vi "Main.vi"() -> ()   [LabVIEW 2018] (continued)
            n155 = Decimal String To Number(string=w532, default (0L)=u32 0 ("默认(0 I32)")) -> (number=w538:u32)  [unwired: 1 in, 1 out]
            n156 = call "S7_Write.vi"("TCP"=w537, "寄存器类型"=w541, "DB #"=u16 20, "写入地址"=u32 58, "数据类型"=w542, "写入数据"=w538) -> ("TCP"=w534:refnum<k5>, "error out"=w533:errorcluster)  [unwired: 7 in, 1 out]
            n157 = Bundle By Name(cluster=w545, "数据保存超时"=w532) -> (w544:T5)
          }
          frame "------------" {
          }
          frame "错误" {
            n158 = Flush Queue(queue=w556) -> ()  [unwired: 1 in, 3 out]
            n159 = Flush Queue(queue=w555) -> ()  [unwired: 1 in, 3 out]
            n160 = call "S7_Close.vi"("TCP Connection Ref"=w559) -> ("error out"=w557:errorcluster)  [unwired: 10 in]
            n161 = call <vilib>:"Clear Errors.vi"("error in (no error)"=w557) -> ()  [unwired: 5 in, 2 out]
          }
          frame "退出" {
            n162 = Release Queue(queue=w567) -> ()  [unwired: 2 in, 3 out]
            n163 = Release Queue(queue=w566) -> ()  [unwired: 2 in, 3 out]
            n164 = call "S7_Close.vi"("TCP Connection Ref"=w565) -> ("error out"=w562:errorcluster)  [unwired: 10 in]
          }
          frame "看门狗" {
            w582 = u8 132 items=["I/O (P)"=128, "Input (I)"=129, "Output (Q)"=130, "Bit Memory (M)"=131, "Data (DB)"=132, "Instance Data (DI)"=133, "Local Data (L)"=134, "Predecessor Local Data (VL)"=135] ("寄存器类型")
            w583 = u16 1 items=["byte", "word", "Dword"] ("数据类型")
            n165 = Unbundle By Name(w575) -> ("看门狗"=w585:string)
            n166 = Decimal String To Number(string=w585) -> (number=w586:i32)  [unwired: 2 in, 1 out]
            n167 = Equal?(x=w586, y=0) -> (x = y?=w588:bool)
            n168 = case shown="假" w588 {
              tunnel: [0 ("y") 1 ("y")] -> w576
              frame False {
              }
              frame True {
              }
            }
            "80" <- w576
            n169 = call "S7_Write.vi"("TCP"=w580, "寄存器类型"=w582, "DB #"=u16 20, "写入地址"=u32 8, "数据类型"=w583, "写入数据"=w576) -> ("TCP"=w573:refnum<k5>, "error out"=w571:errorcluster)  [unwired: 7 in, 1 out]
            n170 = Number To Decimal String(number=w576) -> (decimal integer string=w577:string)  [unwired: 1 in]
            n171 = Bundle By Name(cluster=w575, "看门狗"=w577) -> (w574:T5)
            n172 = disable-structure shown="启用" {
              disable-tunnel: w573 -> [w589 w605]
              disable-tunnel: [w589 w597] -> w572
              disable-tunnel: w571 -> [w590 w596]
              disable-tunnel: [w590 w594] -> w570
              frame Disabled {
              }
              frame Enabled {
                w603 = u16 20 ("DB #")
                w602 = u8 132 items=["I/O (P)"=128, "Input (I)"=129, "Output (Q)"=130, "Bit Memory (M)"=131, "Data (DB)"=132, "Instance Data (DI)"=133, "Local Data (L)"=134, "Predecessor Local Data (VL)"=135] ("寄存器类型")
                w601 = u16 1 items=["byte", "word", "Dword"] ("数据类型")
                n173 = call "S7_Read.vi"("TCP"=w605, "DB #"=w603, "读取长度"=u16 1, "寄存器类型"=w602, "起始地址"=u32 48 ("写入地址"), "数据类型"=w601, "error in"=w596) -> ("TCP"=w604:refnum<k5>, "数据"=w598:u32[], "error out"=w595:errorcluster)  [unwired: 5 in, 1 out]
                n174 = Index Array(array=w598) -> (element=w592:u32)  [unwired: 1 in]
                "80产品型号" <- w592
                n175 = case shown="2" w592 {
                  tunnel: ["未选择" "1" "2"] -> w591
                  frame 0, Default {
                  }
                  frame 1 {
                  }
                  frame 2 {
                  }
                }
                "产品型号" <- w591
                n176 = call "S7_Write.vi"("TCP"=w604, "寄存器类型"=w602, "DB #"=w603, "写入地址"=u32 50, "数据类型"=w601, "写入数据"=w592, "error in"=w595) -> ("TCP"=w597:refnum<k5>, "error out"=w594:errorcluster)  [unwired: 6 in, 1 out]
              }
            }
          }
        }
      }
      n177 = while {
        shift-right: [w6079] -> _
        shift-left: cluster{"Data":string[], "State":T1} {"Data"=[], "State"=enum."PLC通讯初始化"} ("元素") -> [w6080]
        shift-right: [w6088] -> _
        shift-left: w135 -> [w6085]
        shift-right: [w6089] -> _
        shift-left: _ -> [w6086]
        tunnel: w109 -> [w6081]
        tunnel: w116 -> [w6076]
        tunnel: w134 -> [_]
        shift-right: [w6075] -> _
        shift-left: _ -> [w6074]
        stop <- w6077 stop-if-true
        # "OP70"
        n178 = local read "退出"() -> (w6084:bool)
        n179 = Wait (ms)(milliseconds to wait=u32 20 ("等待时间（毫秒）")) -> ()  [unwired: 1 out]
        n180 = call "状态判断.vi"("error IO"=w6085, "退出？"=w6084, "簇 输入"=w6080, "队列输入"=w6081) -> ("簇"=w6083:cluster{"Data":string[], "State":T1})  [unwired: 6 in, 1 out]
        n181 = Unbundle By Name(w6083) -> ("Data"=w6078:string[], "State"=w6082:T1)
        "70_State" <- w6082
        n182 = case shown="\"退出\"" w6082 {
          tunnel: [w6093 w6120 w6142 w6173 w6194 w6245 w6265 w6374 w6402 w6417 refnum<k5> refnum ("TCP") refnum<k5> refnum ("TCP") w6437] -> w6089
          tunnel: [w6094 errorcluster {"status"=FALSE, "code"=0, "source"=""} ("error out") w6141 w6169 w6193 errorcluster {"status"=FALSE, "code"=0, "source"=""} ("error out") w6264 w6321 w6403 errorcluster {"status"=FALSE, "code"=0, "source"=""} ("error out") errorcluster {"status"=FALSE, "code"=0, "source"=""} ("error out") w6429 w6435] -> w6088
          tunnel: w6086 -> [_ w6120 w6143 w6174 w6195 w6245 w6266 w6305 w6405 w6417 w6423 w6430 w6462]
          tunnel: w6081 -> [w6106 _ w6124 _ _ _ w6246 _ _ _ w6419 w6431 _]
          tunnel: [cluster{"Data":string[], "State":T1} {"Data"=[], "State"=enum."读扫码请求"} ("元素") cluster{"Data":string[], "State":T1} {"Data"=[], "State"=enum."读扫码请求"} ("元素") w6131 cluster{"Data":string[], "State":T1} {"Data"=[], "State"=enum."读数据保存请求"} ("元素") cluster{"Data":string[], "State":T1} {"Data"=[], "State"=enum."读数据保存请求"} ("元素") cluster{"Data":string[], "State":T1} {"Data"=[], "State"=enum."读数据保存请求"} ("元素") w6254 cluster{"Data":string[], "State":T1} {"Data"=[], "State"=enum."看门狗"} ("元素") cluster{"Data":string[], "State":T1} {"Data"=[], "State"=enum."看门狗"} ("元素") cluster{"Data":string[], "State":T1} {"Data"=[], "State"=enum."看门狗"} ("元素") cluster{"Data":string[], "State":T1} {"Data"=[], "State"=enum."PLC通讯初始化"} ("元素") cluster{"Data":string[], "State":T1} {"Data"=[], "State"=enum."退出"} ("元素") cluster{"Data":string[], "State":T1} {"Data"=[], "State"=enum."读扫码请求"} ("元素")] -> w6079
          tunnel: w6078 -> [_ _ _ _ w6191 _ _ _ w6404 _ _ _ _]
          tunnel: [FALSE FALSE FALSE FALSE FALSE FALSE FALSE FALSE FALSE FALSE FALSE TRUE FALSE] -> w6077
          tunnel: w6076 -> [_ _ _ _ _ _ _ w6381 _ _ w6420 w6432 _]
          tunnel: [T10 {"扫码超时"="999", "数据保存超时"="999", "看门狗"="999"} w6116 w6123 w6170 w6189 w6241 w6247 w6371 w6398 w6413 w6418 w6427 w6456] -> w6075
          tunnel: w6074 -> [_ w6116 w6123 w6170 w6190 w6241 w6247 w6371 w6399 w6413 w6418 w6427 w6457]
          frame "PLC通讯初始化", Default {
            w6099 = u16 0 items=["byte", "word", "Dword"] ("数据类型")
            w6103 = u8 132 items=["I/O (P)"=128, "Input (I)"=129, "Output (Q)"=130, "Bit Memory (M)"=131, "Data (DB)"=132, "Instance Data (DI)"=133, "Local Data (L)"=134, "Predecessor Local Data (VL)"=135] ("寄存器类型")
            w6114 = u8 0 items=["S7-1200.200.200SMART"=0, "S7-300"=2, "S7-400"=3] ("PLC 系列")
            n183 = Enqueue Element(queue=w6106, element=cluster{"Data":string[], "State":T1} {"Data"=["999"], "State"=enum."扫码回复"} ("元素")) -> (queue out=w6110:refnum<queue>, error out=w6109:errorcluster)  [unwired: 2 in, 1 out]
            n184 = call "S7_Open.vi"("IP 地址"="192.168.0.70", "PLC 系列"=w6114, "超时（MS）"=100) -> ("TCP"=w6096:refnum<k5>, "error out"=w6095:errorcluster)  [unwired: 10 in, 1 out]
            n185 = Unbundle By Name(w6095) -> ("status"=→"ST70通讯状态":bool)
            n186 = Enqueue Element(queue=w6110, element=cluster{"Data":string[], "State":T1} {"Data"=["999"], "State"=enum."数据保存回复"} ("元素"), error in (no error)=w6109) -> ()  [unwired: 1 in, 3 out]
            n187 = call "S7_Read.vi"("TCP"=w6096, "DB #"=u16 20, "读取长度"=u16 17, "寄存器类型"=w6103, "起始地址"=u32 38, "数据类型"=w6099, "error in"=w6095) -> ("TCP"=w6093:refnum<k5>, "数据"=w6098:u32[], "error out"=w6094:errorcluster)  [unwired: 5 in, 1 out]
            n188 = To Unsigned Word Integer(number=w6098) -> (unsigned 16bit integer=w6097:u16[])
            n189 = call "还原为字符串.vi"("输入数组"=w6097) -> ("字符串"=w6091:string)  [unwired: 9 in, 1 out]
            n190 = Match Pattern(string=w6091, regular expression=" " ("正则表达式")) -> (before substring=w6090:string)  [unwired: 1 in, 3 out]
            n191 = local write "70二维码"(w6090) -> ()
          }
          frame "--------------" {
          }
          frame "读扫码请求" {
            w6151 = u16 0 items=["byte", "word", "Dword"] ("数据类型")
            w6153 = u8 132 items=["I/O (P)"=128, "Input (I)"=129, "Output (Q)"=130, "Bit Memory (M)"=131, "Data (DB)"=132, "Instance Data (DI)"=133, "Local Data (L)"=134, "Predecessor Local Data (VL)"=135] ("寄存器类型")
            n192 = call "S7_Read.vi"("TCP"=w6143, "DB #"=u16 20, "读取长度"=u16 1, "寄存器类型"=w6153, "起始地址"=u32 0, "数据类型"=w6151) -> ("TCP"=w6142:refnum<k5>, "数据"=w6148:u32[], "读取成功"=w6121:bool, "error out"=w6141:errorcluster)  [unwired: 6 in]
            n193 = Not(x=w6121) -> (.not. x?=w6122:bool)
            n194 = local write "ST70通讯状态"(w6122) -> ()
            n195 = Index Array(array=w6148, index=0 ("索引")) -> (element=w6146:u32)
            n196 = Number To Boolean Array(number=w6146) -> (Boolean array=w6145:bool[])
            n197 = Index Array(array=w6145, index=0 ("索引")) -> (element=w6130:bool)
            "ST70扫码请求" <- w6130
            n198 = Unbundle By Name(w6123) -> ("扫码超时"=w6125:string)
            n199 = Not Equal?(x=w6125, y="999") -> (x != y?=w6127:bool)
            n200 = call <vilib>:"Boolean Crossing PtByPt.vi"("direction"=enum16{"either", "false-true", "true-false"}."false-true", "input"=w6130) -> ("crossing"=w6137:bool)  [unwired: 1 in]
            n201 = call <vilib>:"Boolean Crossing PtByPt.vi"("direction"=enum16{"either", "false-true", "true-false"}."true-false", "input"=w6130) -> ("crossing"=w6136:bool)  [unwired: 1 in]
            n202 = Not(x=w6127) -> (.not. x?=w6128:bool)
            n203 = call "已用时间15"("Reset"=w6128) -> ("Time has Elapsed"=w6129:bool)  [unwired: 11 in, 7 out]
            n204 = Insert Into Array(array=bool[] [] ("数组"), index=0 ("索引"), new element #1=w6137, new element #2=w6136) -> (w6133:bool[])
            n205 = Boolean Array To Number(Boolean array=w6133) -> (number=w6132:u32)
            n206 = case shown="1" w6132 {
              tunnel: [cluster{"Data":string[], "State":T1} {"Data"=[], "State"=enum."读数据保存请求"} ("元素") w6158 w6162] -> w6131
              tunnel: w6124 -> [_ w6159 w6163]
              frame 0, Default {
              }
              frame 1 {
                w6158 = cluster{"Data":string[], "State":T1} {"Data"=[], "State"=enum."读二维码"} ("元素")
                n207 = Enqueue Element(queue=w6159, element=w6158, timeout in ms (-1)=10 ("超时毫秒(-1)")) -> ()  [unwired: 1 in, 3 out]
              }
              frame 2 {
                w6162 = cluster{"Data":string[], "State":T1} {"Data"=["999"], "State"=enum."扫码回复"} ("元素")
                n208 = Enqueue Element(queue=w6163, element=w6162, timeout in ms (-1)=10 ("超时毫秒(-1)")) -> ()  [unwired: 1 in, 3 out]
              }
            }
            n209 = case shown="真" w6129 {
              tunnel: w6124 -> [_ w6155]
              frame False {
              }
              frame True {
                n210 = Enqueue Element(queue=w6155, element=cluster{"Data":string[], "State":T1} {"Data"=["999"], "State"=enum."扫码回复"} ("元素"), timeout in ms (-1)=10 ("超时毫秒(-1)")) -> ()  [unwired: 1 in, 3 out]
              }
            }
          }
          frame "读二维码" {
            w6179 = u16 0 items=["byte", "word", "Dword"] ("数据类型")
            w6175 = u8 132 items=["I/O (P)"=128, "Input (I)"=129, "Output (Q)"=130, "Bit Memory (M)"=131, "Data (DB)"=132, "Instance Data (DI)"=133, "Local Data (L)"=134, "Predecessor Local Data (VL)"=135] ("寄存器类型")
            n211 = call "S7_Read.vi"("TCP"=w6174, "DB #"=u16 20, "读取长度"=u16 17, "寄存器类型"=w6175, "起始地址"=u32 38, "数据类型"=w6179) -> ("TCP"=w6173:refnum<k5>, "数据"=w6180:u32[], "error out"=w6182:errorcluster)  [unwired: 6 in, 1 out]
            n212 = To Unsigned Word Integer(number=w6180) -> (unsigned 16bit integer=w6181:u16[])
            n213 = call "还原为字符串.vi"("error in (no error)"=w6182, "输入数组"=w6181) -> ("error out"=w6166:errorcluster, "字符串"=w6167:string)  [unwired: 8 in]
            n214 = Match Pattern(string=w6167, regular expression=" " ("正则表达式")) -> (before substring=w6164:string)  [unwired: 1 in, 3 out]
            n215 = flat-sequence {
              tunnel: w6166 -> [w6184]
              tunnel: [w6184] -> w6165
              tunnel: w6164 -> [w6183]
              tunnel: [w6186] -> w6169
              tunnel: w6165 -> [w6185]
              frame #0 {
                "70二维码" <- w6183
              }
              frame #1 {
                n216 = property on="ST70扫码请求(事件)" class="Bool (严格)"(error in=w6185, "Val(Sgnl)"=TRUE ("值(信号)")) -> (error out=w6186:errorcluster)  [unwired: 1 in, 1 out]
              }
            }
          }
          frame "扫码回复" {
            n217 = Array Size(array=w6191) -> (size(s)=w6192:i32)
            n218 = case shown="3, 默认" w6192 {
              tunnel: w6191 -> [w6200 w6233]
              tunnel: w6195 -> [w6199 w6220]
              tunnel: [w6201 w6211] -> w6194
              tunnel: [w6202 w6210] -> w6193
              tunnel: [w6198 w6209] -> w6188
              frame 1 {
                w6205 = u8 132 items=["I/O (P)"=128, "Input (I)"=129, "Output (Q)"=130, "Bit Memory (M)"=131, "Data (DB)"=132, "Instance Data (DI)"=133, "Local Data (L)"=134, "Predecessor Local Data (VL)"=135] ("寄存器类型")
                w6204 = u16 1 items=["byte", "word", "Dword"] ("数据类型")
                n219 = Index Array(array=w6200) -> (element=w6198:string)  [unwired: 1 in]
                n220 = Decimal String To Number(string=w6198, default (0L)=u32 0 ("默认(0 I32)")) -> (number=w6208:u32)  [unwired: 1 in, 1 out]
                n221 = call "S7_Write.vi"("TCP"=w6199, "寄存器类型"=w6205, "DB #"=u16 20, "写入地址"=u32 2, "数据类型"=w6204, "写入数据"=w6208) -> ("TCP"=w6201:refnum<k5>, "error out"=w6202:errorcluster)  [unwired: 7 in, 1 out]
              }
              frame 3, Default {
                w6223 = u8 132 items=["I/O (P)"=128, "Input (I)"=129, "Output (Q)"=130, "Bit Memory (M)"=131, "Data (DB)"=132, "Instance Data (DI)"=133, "Local Data (L)"=134, "Predecessor Local Data (VL)"=135] ("寄存器类型")
                w6222 = u16 1 items=["byte", "word", "Dword"] ("数据类型")
                w6230 = u8 132 items=["I/O (P)"=128, "Input (I)"=129, "Output (Q)"=130, "Bit Memory (M)"=131, "Data (DB)"=132, "Instance Data (DI)"=133, "Local Data (L)"=134, "Predecessor Local Data (VL)"=135] ("寄存器类型")
                w6231 = u16 1 items=["byte", "word", "Dword"] ("数据类型")
                w6237 = u8 132 items=["I/O (P)"=128, "Input (I)"=129, "Output (Q)"=130, "Bit Memory (M)"=131, "Data (DB)"=132, "Instance Data (DI)"=133, "Local Data (L)"=134, "Predecessor Local Data (VL)"=135] ("寄存器类型")
                w6236 = u16 1 items=["byte", "word", "Dword"] ("数据类型")
                n222 = Index Array(array=w6233) -> (element #1=w6209:string, element #2=w6216:string, element #3=w6215:string)  [unwired: 3 in]
                n223 = Equal?(x=w6215, y="OK") -> (x = y?=w6213:bool)
                n224 = Decimal String To Number(string=w6216, default (0L)=u32 0 ("默认(0 I32)")) -> (number=w6217:u32)  [unwired: 1 in, 1 out]
                n225 = case shown="假" w6213 {
                  tunnel: [u32 2 ("写入数据") u32 1 ("写入数据")] -> w6212
                  frame False {
                  }
                  frame True {
                  }
                }
                n226 = call "S7_Write.vi"("TCP"=w6220, "寄存器类型"=w6237, "DB #"=u16 20, "写入地址"=u32 8, "数据类型"=w6236, "写入数据"=w6217) -> ("TCP"=w6227:refnum<k5>, "error out"=w6228:errorcluster)  [unwired: 7 in, 1 out]
                n227 = call "S7_Write.vi"("TCP"=w6227, "寄存器类型"=w6230, "DB #"=u16 20, "写入地址"=u32 10, "数据类型"=w6231, "写入数据"=w6212, "error in"=w6228) -> ("TCP"=w6219:refnum<k5>, "error out"=w6218:errorcluster)  [unwired: 6 in, 1 out]
                n228 = Decimal String To Number(string=w6209, default (0L)=u32 0 ("默认(0 I32)")) -> (number=w6226:u32)  [unwired: 1 in, 1 out]
                n229 = call "S7_Write.vi"("TCP"=w6219, "寄存器类型"=w6223, "DB #"=u16 20, "写入地址"=u32 2, "数据类型"=w6222, "写入数据"=w6226, "error in"=w6218) -> ("TCP"=w6211:refnum<k5>, "error out"=w6210:errorcluster)  [unwired: 6 in, 1 out]
              }
            }
            "扫码请求回复70" <- w6188
            n230 = Bundle By Name(cluster=w6190, "扫码超时"=w6188) -> (w6189:T10)
          }
          frame "-------------" {
          }
          frame "读数据保存请求" {
            w6274 = u16 0 items=["byte", "word", "Dword"] ("数据类型")
            w6276 = u8 132 items=["I/O (P)"=128, "Input (I)"=129, "Output (Q)"=130, "Bit Memory (M)"=131, "Data (DB)"=132, "Instance Data (DI)"=133, "Local Data (L)"=134, "Predecessor Local Data (VL)"=135] ("寄存器类型")
            n231 = call "S7_Read.vi"("TCP"=w6266, "DB #"=u16 20, "读取长度"=u16 1, "寄存器类型"=w6276, "起始地址"=u32 0, "数据类型"=w6274) -> ("TCP"=w6265:refnum<k5>, "数据"=w6271:u32[], "error out"=w6264:errorcluster)  [unwired: 6 in, 1 out]
            n232 = Index Array(array=w6271, index=0 ("索引")) -> (element=w6269:u32)
            n233 = Number To Boolean Array(number=w6269) -> (Boolean array=w6268:bool[])
            n234 = Index Array(array=w6268, index #1=1 ("索引")) -> (element #1=w6253:bool)  [unwired: 1 in, 1 out]
            "ST70数据读取" <- w6253
            n235 = Unbundle By Name(w6247) -> ("数据保存超时"=w6248:string)
            n236 = Not Equal?(x=w6248, y="999") -> (x != y?=w6250:bool)
            n237 = Not(x=w6250) -> (.not. x?=w6251:bool)
            n238 = call <vilib>:"Boolean Crossing PtByPt.vi"("direction"=enum16{"either", "false-true", "true-false"}."false-true", "input"=w6253) -> ("crossing"=w6257:bool)  [unwired: 1 in]
            n239 = call <vilib>:"Boolean Crossing PtByPt.vi"("direction"=enum16{"either", "false-true", "true-false"}."true-false", "input"=w6253) -> ("crossing"=w6258:bool)  [unwired: 1 in]
            n240 = call "已用时间16"("Reset"=w6251) -> ("Time has Elapsed"=w6252:bool)  [unwired: 11 in, 7 out]
            n241 = Insert Into Array(array=bool[] [] ("数组"), index=0 ("索引"), new element #1=w6257, new element #2=w6258) -> (w6261:bool[])
            n242 = Boolean Array To Number(Boolean array=w6261) -> (number=w6262:u32)
            n243 = case shown="0, 默认" w6262 {
              tunnel: [cluster{"Data":string[], "State":T1} {"Data"=[], "State"=enum."看门狗"} ("元素") w6282 w6284] -> w6254
              tunnel: w6246 -> [_ w6283 w6285]
              frame 0, Default {
              }
              frame 1 {
                w6282 = cluster{"Data":string[], "State":T1} {"Data"=[], "State"=enum."读数据"} ("元素")
                n244 = Enqueue Element(queue=w6283, element=w6282, timeout in ms (-1)=10 ("超时毫秒(-1)")) -> ()  [unwired: 1 in, 3 out]
              }
              frame 2 {
                w6284 = cluster{"Data":string[], "State":T1} {"Data"=["999"], "State"=enum."数据保存回复"} ("元素")
                n245 = Enqueue Element(queue=w6285, element=w6284, timeout in ms (-1)=10 ("超时毫秒(-1)")) -> ()  [unwired: 1 in, 3 out]
              }
            }
            n246 = case shown="真" w6252 {
              tunnel: w6246 -> [_ w6278]
              frame False {
              }
              frame True {
                n247 = Enqueue Element(queue=w6278, element=cluster{"Data":string[], "State":T1} {"Data"=["999"], "State"=enum."数据保存回复"} ("元素"), timeout in ms (-1)=10 ("超时毫秒(-1)")) -> ()  [unwired: 1 in, 3 out]
              }
            }
          }
          frame "读数据" {
            w6302 = u16 2 items=["byte", "word", "Dword"] ("数据类型")
            w6300 = u8 132 items=["I/O (P)"=128, "Input (I)"=129, "Output (Q)"=130, "Bit Memory (M)"=131, "Data (DB)"=132, "Instance Data (DI)"=133, "Local Data (L)"=134, "Predecessor Local Data (VL)"=135] ("寄存器类型")
            w6306 = u16 0 items=["byte", "word", "Dword"] ("数据类型")
            w6308 = u8 132 items=["I/O (P)"=128, "Input (I)"=129, "Output (Q)"=130, "Bit Memory (M)"=131, "Data (DB)"=132, "Instance Data (DI)"=133, "Local Data (L)"=134, "Predecessor Local Data (VL)"=135] ("寄存器类型")
            w6357 = u16 2 items=["byte", "word", "Dword"] ("数据类型")
            w6355 = u8 132 items=["I/O (P)"=128, "Input (I)"=129, "Output (Q)"=130, "Bit Memory (M)"=131, "Data (DB)"=132, "Instance Data (DI)"=133, "Local Data (L)"=134, "Predecessor Local Data (VL)"=135] ("寄存器类型")
            w6363 = u16 0 items=["byte", "word", "Dword"] ("数据类型")
            w6365 = u8 132 items=["I/O (P)"=128, "Input (I)"=129, "Output (Q)"=130, "Bit Memory (M)"=131, "Data (DB)"=132, "Instance Data (DI)"=133, "Local Data (L)"=134, "Predecessor Local Data (VL)"=135] ("寄存器类型")
            w6392 = u16 1 items=["byte", "word", "Dword"] ("数据类型")
            w6388 = u8 132 items=["I/O (P)"=128, "Input (I)"=129, "Output (Q)"=130, "Bit Memory (M)"=131, "Data (DB)"=132, "Instance Data (DI)"=133, "Local Data (L)"=134, "Predecessor Local Data (VL)"=135] ("寄存器类型")
            n248 = call "S7_Read.vi"("TCP"=w6305, "DB #"=u16 20, "读取长度"=u16 1, "寄存器类型"=w6308, "起始地址"=u32 0, "数据类型"=w6306) -> ("TCP"=w6297:refnum<k5>, "数据"=w6315:u32[], "error out"=w6296:errorcluster)  [unwired: 6 in, 1 out]
            n249 = Index Array(array=w6315, index=0 ("索引")) -> (element=w6314:u32)
            n250 = Number To Boolean Array(number=w6314) -> (Boolean array=w6313:bool[])
            n251 = call "S7_Read.vi"("TCP"=w6297, "DB #"=u16 20, "读取长度"=u16 3, "寄存器类型"=w6300, "起始地址"=u32 90, "数据类型"=w6302, "error in"=w6296) -> ("TCP"=w6294:refnum<k5>, "数据"=w6293:u32[], "error out"=w6295:errorcluster)  [unwired: 5 in, 1 out]
            n252 = Index Array(array=w6313, index=3 ("索引")) -> (element=w6311:bool)
            n253 = Equal?(x=w6311, y=TRUE) -> (x = y?=w6312:bool)
            n254 = Number To Decimal String(number=w6293) -> (decimal integer string=w6292:string[])  [unwired: 1 in]
            n255 = Index Array(array=w6292) -> (element #1=w6291:string, element #2=w6290:string, element #3=w6289:string)  [unwired: 3 in]
            n256 = case shown="假" w6312 {
              tunnel: [" " "Y"] -> w6304
              frame False {
              }
              frame True {
              }
            }
            n257 = call "S7_Read.vi"("TCP"=w6294, "DB #"=u16 20, "读取长度"=u16 21, "寄存器类型"=w6365, "起始地址"=u32 56, "数据类型"=w6363, "error in"=w6295) -> ("TCP"=w6352:refnum<k5>, "数据"=w6368:u32[], "error out"=w6351:errorcluster)  [unwired: 5 in, 1 out]
            "数据" <- w6368
            n258 = To Unsigned Word Integer(number=w6368) -> (unsigned 16bit integer=w6369:u16[])
            n259 = call "还原为字符串.vi"("输入数组"=w6369) -> ("字符串"=w6360:string)  [unwired: 9 in, 1 out]
            n260 = call "S7_Read.vi"("TCP"=w6352, "DB #"=u16 20, "读取长度"=u16 6, "寄存器类型"=w6355, "起始地址"=u32 12, "数据类型"=w6357, "error in"=w6351) -> ("TCP"=w6350:refnum<k5>, "数据"=w6348:u32[], "error out"=w6349:errorcluster)  [unwired: 5 in, 1 out]
            n261 = Index Array(array=w6348) -> (element #1=w6345:u32, element #2=w6347:u32, element #3=w6342:u32, element #4=w6341:u32, element #5=w6334:u32, element #6=w6333:u32)  [unwired: 6 in]
            n262 = call "S7_Read.vi"("TCP"=w6350, "DB #"=u16 20, "读取长度"=u16 1, "寄存器类型"=w6388, "起始地址"=u32 6, "数据类型"=w6392, "error in"=w6349) -> ("TCP"=w6374:refnum<k5>, "数据"=w6385:u32[], "error out"=w6373:errorcluster)  [unwired: 5 in, 1 out]
            n263 = Divide(x=w6347, y=u32 100) -> (x/y=w6344:dbl)
            n264 = Divide(x=w6334, y=u32 100) -> (x/y=w6339:dbl)
            n265 = Divide(x=w6333, y=u32 100) -> (x/y=w6336:dbl)
            n266 = Index Array(array=w6385) -> (element=w6372:u32)  [unwired: 1 in]
            n267 = Number To Decimal String(number=w6345) -> (decimal integer string=w6329:string)  [unwired: 1 in]
            n268 = Number To Fractional String(number=w6344, precision (6)=i16 2 ("精度(6)")) -> (F-format string=w6326:string)  [unwired: 2 in]
            n269 = Number To Decimal String(number=w6342) -> (decimal integer string=w6328:string)  [unwired: 1 in]
            n270 = Number To Decimal String(number=w6341) -> (decimal integer string=w6327:string)  [unwired: 1 in]
            n271 = Number To Fractional String(number=w6339, precision (6)=i16 2 ("精度(6)")) -> (F-format string=w6325:string)  [unwired: 2 in]
            n272 = String Subset(string=w6360, offset (0)=0 ("偏移量(0)"), length (rest)=20 ("长度（剩余）")) -> (substring=w6319:string)
            n273 = String Subset(string=w6360, offset (0)=20 ("偏移量(0)"), length (rest)=1 ("长度（剩余）")) -> (substring=w6330:string)
            n274 = Number To Fractional String(number=w6336, precision (6)=i16 2 ("精度(6)")) -> (F-format string=w6324:string)  [unwired: 2 in]
            n275 = Equal?(x=w6372, y=u32 1) -> (x = y?=w6383:bool)
            n276 = local read "ST70 Shaft Seal 5024366"() -> (w6323:string)
            n277 = case shown="真" w6383 {
              tunnel: ["NG" "OK"] -> w6370
              frame False {
              }
              frame True {
              }
            }
            n278 = Format Date/Time String(time format string (%c)="%Y-%m-%d" ("时间格式字符串(%c)")) -> (date/time string=w6376:string)  [unwired: 2 in]
            n279 = Get Date/Time String() -> (time string=w6375:string)  [unwired: 3 in, 1 out]
            n280 = String Subset(string=w6319, offset (0)=0 ("偏移量(0)"), length (rest)=17 ("长度（剩余）")) -> (substring=w6316:string)
            "刻印码" <- w6316
            "刻印码 16" <- w6316
            n281 = Insert Into Array(array=string[] [] ("数组"), index=0 ("索引"), new element #1="70" ("新元素/子数组"), new element #2=w6370, new element #3=w6376, new element #4=w6375, new element #5=w6370, new element #6=w6316, new element #7=w6330, new element #8=w6329, new element #9=w6328, new element #10=w6327, new element #11=w6326, new element #12=w6325, new element #13=w6324, new element #14=w6323, new element #15=w6304, new element #16=w6291, new element #17=w6290, new element #18=w6289) -> (w6382:string[])
            n282 = Enqueue Element(queue=w6381, element=w6382, error in (no error)=w6373) -> (error out=w6331:errorcluster)  [unwired: 1 in, 2 out]
            n283 = property on="ST70数据读取(事件)" class="Bool (严格)"(error in=w6331, "Val(Sgnl)"=TRUE ("值(信号)")) -> (error out=w6322:errorcluster)  [unwired: 1 in, 1 out]
            n284 = property on="OP70画曲线" class="Bool (严格)"(error in=w6322, "Val(Sgnl)"=TRUE ("值(信号)")) -> (error out=w6321:errorcluster)  [unwired: 1 in, 1 out]
          }
          frame "数据保存回复" {
            w6410 = u8 132 items=["I/O (P)"=128, "Input (I)"=129, "Output (Q)"=130, "Bit Memory (M)"=131, "Data (DB)"=132, "Instance Data (DI)"=133, "Local Data (L)"=134, "Predecessor Local Data (VL)"=135] ("寄存器类型")
            w6411 = u16 1 items=["byte", "word", "Dword"] ("数据类型")
            n285 = Index Array(array=w6404, index=0 ("索引")) -> (element=w6397:string)
            "数据保存请求回复70" <- w6397
            n286 = Decimal String To Number(string=w6397, default (0L)=u32 0 ("默认(0 I32)")) -> (number=w6406:u32)  [unwired: 1 in, 1 out]
            n287 = call "S7_Write.vi"("TCP"=w6405, "寄存器类型"=w6410, "DB #"=u16 20, "写入地址"=u32 4, "数据类型"=w6411, "写入数据"=w6406) -> ("TCP"=w6402:refnum<k5>, "error out"=w6403:errorcluster)  [unwired: 7 in, 1 out]
            n288 = Bundle By Name(cluster=w6399, "数据保存超时"=w6397) -> (w6398:T10)
          }
          frame "-----------------" {
          }
          frame "错误" {
            n289 = Flush Queue(queue=w6420) -> ()  [unwired: 1 in, 3 out]
            n290 = Flush Queue(queue=w6419) -> ()  [unwired: 1 in, 3 out]
            n291 = call "S7_Close.vi"("TCP Connection Ref"=w6423) -> ("error out"=w6421:errorcluster)  [unwired: 10 in]
            n292 = call <vilib>:"Clear Errors.vi"("error in (no error)"=w6421) -> ()  [unwired: 5 in, 2 out]
          }
          frame "退出" {
            n293 = Release Queue(queue=w6432) -> ()  [unwired: 2 in, 3 out]
            n294 = Release Queue(queue=w6431) -> ()  [unwired: 2 in, 3 out]
            n295 = call "S7_Close.vi"("TCP Connection Ref"=w6430) -> ("error out"=w6429:errorcluster)  [unwired: 10 in]
          }
          frame "看门狗" {
            w6446 = u8 132 items=["I/O (P)"=128, "Input (I)"=129, "Output (Q)"=130, "Bit Memory (M)"=131, "Data (DB)"=132, "Instance Data (DI)"=133, "Local Data (L)"=134, "Predecessor Local Data (VL)"=135] ("寄存器类型")
            w6445 = u16 1 items=["byte", "word", "Dword"] ("数据类型")
            w6464 = u8 132 items=["I/O (P)"=128, "Input (I)"=129, "Output (Q)"=130, "Bit Memory (M)"=131, "Data (DB)"=132, "Instance Data (DI)"=133, "Local Data (L)"=134, "Predecessor Local Data (VL)"=135] ("寄存器类型")
            w6465 = u16 1 items=["byte", "word", "Dword"] ("数据类型")
            n296 = Unbundle By Name(w6457) -> ("看门狗"=w6467:string)
            n297 = Decimal String To Number(string=w6467) -> (number=w6468:i32)  [unwired: 2 in, 1 out]
            n298 = Equal?(x=w6468, y=0) -> (x = y?=w6470:bool)
            n299 = case shown="假" w6470 {
              tunnel: [0 ("y") 1 ("y")] -> w6458
              frame False {
              }
              frame True {
              }
            }
            "70" <- w6458
            n300 = Format Date/Time String(time format string (%c)="%Y%m%d") -> (date/time string=w6451:string)  [unwired: 2 in]
            n301 = call "S7_Write.vi"("TCP"=w6462, "寄存器类型"=w6464, "DB #"=u16 20, "写入地址"=u32 36, "数据类型"=w6465, "写入数据"=w6458) -> ("TCP"=w6455:refnum<k5>, "error out"=w6454:errorcluster)  [unwired: 7 in, 1 out]
            n302 = Number To Decimal String(number=w6458) -> (decimal integer string=w6459:string)  [unwired: 1 in]
            n303 = for {
              N: 8 -> [_]
              tunnel: w6451 -> [w6498]
              shift-right: [w6496] -> _
              shift-left: 0 -> [w6497]
              tunnel: [w6491] -> w6449 mode=indexing
              n304 = String Subset(string=w6498, offset (0)=w6497, length (rest)=1 ("长度（剩余）")) -> (substring=w6494:string)
              n305 = Increment(x=w6497) -> (x+1=w6496:i32)
              n306 = String To Byte Array(string=w6494) -> (unsigned byte array=w6493:u8[])
              n307 = Index Array(array=w6493, index=0 ("索引")) -> (element=w6491:u8)
            }
            n308 = Bundle By Name(cluster=w6457, "看门狗"=w6459) -> (w6456:T10)
            n309 = for {
              shift-right: [w6485] -> w6443
              shift-left: w6455 -> [w6487]
              shift-right: [w6484] -> w6442
              shift-left: w6454 -> [w6486]
              tunnel: w6449 -> [w6483] mode=indexing
              tunnel: u32[] [78, 79, 80, 81, 82, 83, 84, 85] -> [w6482] mode=indexing
              w6489 = u8 132 items=["I/O (P)"=128, "Input (I)"=129, "Output (Q)"=130, "Bit Memory (M)"=131, "Data (DB)"=132, "Instance Data (DI)"=133, "Local Data (L)"=134, "Predecessor Local Data (VL)"=135] ("寄存器类型")
              w6488 = u16 0 items=["byte", "word", "Dword"] ("数据类型")
              n310 = call "S7_Write.vi"("TCP"=w6487, "寄存器类型"=w6489, "DB #"=u16 20, "写入地址"=w6482, "数据类型"=w6488, "写入数据"=w6483, "error in"=w6486) -> ("TCP"=w6485:refnum<k5>, "error out"=w6484:errorcluster)  [unwired: 6 in, 1 out]
            }
            n311 = Format Date/Time String(time format string (%c)="%j") -> (date/time string=w6440:string)  [unwired: 2 in]
            n312 = Decimal String To Number(string=w6440) -> (number=w6439:i32)  [unwired: 2 in, 1 out]
            n313 = call "S7_Write.vi"("TCP"=w6443, "寄存器类型"=w6446, "DB #"=u16 20, "写入地址"=u32 102, "数据类型"=w6445, "写入数据"=w6439, "error in"=w6442) -> ("TCP"=w6438:refnum<k5>, "error out"=w6436:errorcluster)  [unwired: 6 in, 1 out]
            n314 = disable-structure shown="启用" {
              disable-tunnel: w6438 -> [w6471 w6475]
              disable-tunnel: [w6471 w6478] -> w6437
              disable-tunnel: w6436 -> [w6472 w6476]
              disable-tunnel: [w6472 w6477] -> w6435
              frame Disabled {
              }
              frame Enabled {
                w6480 = u8 132 items=["I/O (P)"=128, "Input (I)"=129, "Output (Q)"=130, "Bit Memory (M)"=131, "Data (DB)"=132, "Instance Data (DI)"=133, "Local Data (L)"=134, "Predecessor Local Data (VL)"=135] ("寄存器类型")
                w6474 = u16 1 items=["byte", "word", "Dword"] ("数据类型")
                n315 = local read "80产品型号"() -> (w6473:u32)
                n316 = call "S7_Write.vi"("TCP"=w6475, "寄存器类型"=w6480, "DB #"=u16 20, "写入地址"=u32 104, "数据类型"=w6474, "写入数据"=w6473, "error in"=w6476) -> ("TCP"=w6478:refnum<k5>, "error out"=w6477:errorcluster)  [unwired: 6 in, 1 out]
              }
            }
          }
        }
      }
      n317 = while {
        shift-right: [w4851] -> _
        shift-left: cluster{"Data":string[], "State":T1} {"Data"=[], "State"=enum."PLC通讯初始化"} ("元素") -> [w4852]
        shift-right: [w4860] -> _
        shift-left: w139 -> [w4857]
        shift-right: [w4861] -> _
        shift-left: _ -> [w4858]
        tunnel: w137 -> [w4853]
        tunnel: w136 -> [w4848]
        tunnel: w138 -> [_]
        shift-right: [w4847] -> _
        shift-left: _ -> [w4846]
        stop <- w4849 stop-if-true
        # "OP50"
        n318 = local read "退出"() -> (w4856:bool)
        n319 = Wait (ms)(milliseconds to wait=u32 20 ("等待时间（毫秒）")) -> ()  [unwired: 1 out]
        n320 = call "状态判断.vi"("error IO"=w4857, "退出？"=w4856, "簇 输入"=w4852, "队列输入"=w4853) -> ("簇"=w4855:cluster{"Data":string[], "State":T1})  [unwired: 6 in, 1 out]
        n321 = Unbundle By Name(w4855) -> ("Data"=w4850:string[], "State"=w4854:T1)
        "50_State" <- w4854
        n322 = case shown="\"扫码回复2\"" w4854 {
          tunnel: [w4869 w4910 w4932 w4963 w4984 w5035 w5055 w5118 w5146 w5161 refnum<k5> refnum ("TCP") refnum<k5> refnum ("TCP") w5183 w5208 w5250 w5270 w5321 w5332 w5366 w5401 w5414 w5420] -> w4861
          tunnel: [w4868 errorcluster {"status"=FALSE, "code"=0, "source"=""} ("error out") w4931 w4960 w4983 errorcluster {"status"=FALSE, "code"=0, "source"=""} ("error out") w5054 w5112 w5147 errorcluster {"status"=FALSE, "code"=0, "source"=""} ("error out") errorcluster {"status"=FALSE, "code"=0, "source"=""} ("error out") w5173 errorcluster {"status"=FALSE, "code"=0, "source"=""} ("error out") w5207 w5247 w5269 errorcluster {"status"=FALSE, "code"=0, "source"=""} ("error out") w5331 w5371 w5400 errorcluster {"status"=FALSE, "code"=0, "source"=""} ("error out") w5418] -> w4860
          tunnel: w4858 -> [_ w4910 w4933 w4964 w4985 w5035 w5056 w5097 w5149 w5161 w5167 w5174 w5183 w5186 w5251 w5271 w5321 w5333 w5368 w5403 w5414 w5451]
          tunnel: w4853 -> [w4896 _ w4913 _ _ _ w5036 _ _ _ w5163 w5175 _ w5199 _ _ _ w5322 _ _ _ _]
          tunnel: [cluster{"Data":string[], "State":T1} {"Data"=[], "State"=enum."读扫码请求"} ("元素") cluster{"Data":string[], "State":T1} {"Data"=[], "State"=enum."读扫码请求"} ("元素") w4921 cluster{"Data":string[], "State":T1} {"Data"=[], "State"=enum."读数据保存请求"} ("元素") cluster{"Data":string[], "State":T1} {"Data"=[], "State"=enum."读数据保存请求"} ("元素") cluster{"Data":string[], "State":T1} {"Data"=[], "State"=enum."读数据保存请求"} ("元素") w5044 cluster{"Data":string[], "State":T1} {"Data"=[], "State"=enum."读扫码请求2"} ("元素") cluster{"Data":string[], "State":T1} {"Data"=[], "State"=enum."读扫码请求2"} ("元素") cluster{"Data":string[], "State":T1} {"Data"=[], "State"=enum."读扫码请求2"} ("元素") cluster{"Data":string[], "State":T1} {"Data"=[], "State"=enum."PLC通讯初始化"} ("元素") cluster{"Data":string[], "State":T1} {"Data"=[], "State"=enum."退出"} ("元素") cluster{"Data":string[], "State":T1} {"Data"=[], "State"=enum."读扫码请求2"} ("元素") w5206 cluster{"Data":string[], "State":T1} {"Data"=[], "State"=enum."读数据保存请求2"} ("元素") cluster{"Data":string[], "State":T1} {"Data"=[], "State"=enum."读数据保存请求2"} ("元素") cluster{"Data":string[], "State":T1} {"Data"=[], "State"=enum."读数据保存请求2"} ("元素") w5330 cluster{"Data":string[], "State":T1} {"Data"=[], "State"=enum."看门狗"} ("元素") cluster{"Data":string[], "State":T1} {"Data"=[], "State"=enum."看门狗"} ("元素") cluster{"Data":string[], "State":T1} {"Data"=[], "State"=enum."看门狗"} ("元素") cluster{"Data":string[], "State":T1} {"Data"=[], "State"=enum."读扫码请求"} ("元素")] -> w4851
          tunnel: w4850 -> [_ _ _ _ w4982 _ _ _ w5148 _ _ _ _ _ _ w5272 _ _ _ w5402 _ _]
          tunnel: [FALSE FALSE FALSE FALSE FALSE FALSE FALSE FALSE FALSE FALSE FALSE TRUE FALSE FALSE FALSE FALSE FALSE FALSE FALSE FALSE FALSE FALSE] -> w4849
          tunnel: w4848 -> [_ _ _ _ _ _ _ w5117 _ _ w5164 w5176 _ _ _ _ _ _ _ _ _ _]
          tunnel: [T7 {"扫码超时1"="999", "数据保存超时1"="999", "扫码超时2"="999", "数据保存超时2"="999", "看门狗"="999", "扫码超时3"="999", "数据保存超时3"="999", "条码"="", "次数"=0} w4906 w4914 w4959 w4978 w5031 w5037 w5114 w5142 w5157 w5162 w5171 w5179 w5187 w5246 w5265 w5317 w5323 w5369 w5396 w5415 w5445] -> w4847
          tunnel: w4846 -> [_ w4906 w4914 w4959 w4979 w5031 w5037 w5114 w5143 w5157 w5162 w5171 w5179 w5188 w5246 w5266 w5317 w5323 w5369 w5397 w5415 w5446]
          frame "PLC通讯初始化", Default {
            w4878 = u16 0 items=["byte", "word", "Dword"] ("数据类型")
            w4874 = u8 132 items=["I/O (P)"=128, "Input (I)"=129, "Output (Q)"=130, "Bit Memory (M)"=131, "Data (DB)"=132, "Instance Data (DI)"=133, "Local Data (L)"=134, "Predecessor Local Data (VL)"=135] ("寄存器类型")
            w4885 = u16 0 items=["byte", "word", "Dword"] ("数据类型")
            w4881 = u8 132 items=["I/O (P)"=128, "Input (I)"=129, "Output (Q)"=130, "Bit Memory (M)"=131, "Data (DB)"=132, "Instance Data (DI)"=133, "Local Data (L)"=134, "Predecessor Local Data (VL)"=135] ("寄存器类型")
            w4904 = u8 0 items=["S7-1200.200.200SMART"=0, "S7-300"=2, "S7-400"=3] ("PLC 系列")
            n323 = Enqueue Element(queue=w4896, element=cluster{"Data":string[], "State":T1} {"Data"=["999"], "State"=enum."扫码回复"} ("元素")) -> (queue out=w4900:refnum<queue>, error out=w4899:errorcluster)  [unwired: 2 in, 1 out]
            n324 = call "S7_Open.vi"("IP 地址"="192.168.0.50", "PLC 系列"=w4904, "超时（MS）"=100) -> ("TCP"=w4871:refnum<k5>, "error out"=w4870:errorcluster)  [unwired: 10 in, 1 out]
            n325 = Enqueue Element(queue=w4900, element=cluster{"Data":string[], "State":T1} {"Data"=["999"], "State"=enum."数据保存回复"} ("元素"), error in (no error)=w4899) -> (queue out=w4890:refnum<queue>, error out=w4889:errorcluster)  [unwired: 1 in, 1 out]
            n326 = Unbundle By Name(w4870) -> ("status"=→"ST50通讯状态":bool)
            n327 = Enqueue Element(queue=w4890, element=cluster{"Data":string[], "State":T1} {"Data"=["999"], "State"=enum."扫码回复2"} ("元素"), error in (no error)=w4889) -> (queue out=w4893:refnum<queue>, error out=w4894:errorcluster)  [unwired: 1 in, 1 out]
            n328 = Enqueue Element(queue=w4893, element=cluster{"Data":string[], "State":T1} {"Data"=["999"], "State"=enum."数据保存回复2"} ("元素"), error in (no error)=w4894) -> ()  [unwired: 1 in, 3 out]
            n329 = call "S7_Read.vi"("TCP"=w4871, "DB #"=u16 20, "读取长度"=u16 17, "寄存器类型"=w4881, "起始地址"=u32 24, "数据类型"=w4885, "error in"=w4870) -> ("TCP"=w4873:refnum<k5>, "数据"=w4886:u32[], "error out"=w4872:errorcluster)  [unwired: 5 in, 1 out]
            n330 = To Unsigned Word Integer(number=w4886) -> (unsigned 16bit integer=w4887:u16[])
            n331 = call "还原为字符串.vi"("输入数组"=w4887) -> ("字符串"=w4866:string)  [unwired: 9 in, 1 out]
            n332 = Match Pattern(string=w4866, regular expression=" " ("正则表达式")) -> (before substring=w4865:string)  [unwired: 1 in, 3 out]
            n333 = local write "502二维码"(w4865) -> ()
            n334 = call "S7_Read.vi"("TCP"=w4873, "DB #"=u16 20, "读取长度"=u16 17, "寄存器类型"=w4874, "起始地址"=u32 42, "数据类型"=w4878, "error in"=w4872) -> ("TCP"=w4869:refnum<k5>, "数据"=w4879:u32[], "error out"=w4868:errorcluster)  [unwired: 5 in, 1 out]
            n335 = To Unsigned Word Integer(number=w4879) -> (unsigned 16bit integer=w4880:u16[])
            n336 = call "还原为字符串.vi"("输入数组"=w4880) -> ("字符串"=w4863:string)  [unwired: 9 in, 1 out]
            n337 = Match Pattern(string=w4863, regular expression=" " ("正则表达式")) -> (before substring=w4862:string)  [unwired: 1 in, 3 out]
            n338 = local write "503二维码"(w4862) -> ()
          }
          frame "--------------" {
          }
          frame "读扫码请求" {
            w4941 = u16 0 items=["byte", "word", "Dword"] ("数据类型")
            w4943 = u8 132 items=["I/O (P)"=128, "Input (I)"=129, "Output (Q)"=130, "Bit Memory (M)"=131, "Data (DB)"=132, "Instance Data (DI)"=133, "Local Data (L)"=134, "Predecessor Local Data (VL)"=135] ("寄存器类型")
            n339 = call "S7_Read.vi"("TCP"=w4933, "DB #"=u16 20, "读取长度"=u16 1, "寄存器类型"=w4943, "起始地址"=u32 0, "数据类型"=w4941) -> ("TCP"=w4932:refnum<k5>, "数据"=w4938:u32[], "读取成功"=w4911:bool, "error out"=w4931:errorcluster)  [unwired: 6 in]
            n340 = Not(x=w4911) -> (.not. x?=w4912:bool)
            n341 = Index Array(array=w4938, index=0 ("索引")) -> (element=w4936:u32)
            n342 = local write "ST50通讯状态"(w4912) -> ()
            n343 = Number To Boolean Array(number=w4936) -> (Boolean array=w4935:bool[])
            n344 = Index Array(array=w4935, index=0 ("索引")) -> (element=w4920:bool)
            "ST501扫码请求" <- w4920
            n345 = Unbundle By Name(w4914) -> ("扫码超时1"=w4915:string)
            n346 = Not Equal?(x=w4915, y="999") -> (x != y?=w4917:bool)
            n347 = Not(x=w4917) -> (.not. x?=w4918:bool)
            n348 = call <vilib>:"Boolean Crossing PtByPt.vi"("direction"=enum16{"either", "false-true", "true-false"}."false-true", "input"=w4920) -> ("crossing"=w4927:bool)  [unwired: 1 in]
            n349 = call <vilib>:"Boolean Crossing PtByPt.vi"("direction"=enum16{"either", "false-true", "true-false"}."true-false", "input"=w4920) -> ("crossing"=w4926:bool)  [unwired: 1 in]
            n350 = call "已用时间11"("Reset"=w4918) -> ("Time has Elapsed"=w4919:bool)  [unwired: 11 in, 7 out]
            n351 = Insert Into Array(array=bool[] [] ("数组"), index=0 ("索引"), new element #1=w4927, new element #2=w4926) -> (w4923:bool[])
            n352 = Boolean Array To Number(Boolean array=w4923) -> (number=w4922:u32)
            n353 = case shown="真" w4919 {
              tunnel: w4913 -> [_ w4945]
              frame False {
              }
              frame True {
                n354 = Enqueue Element(queue=w4945, element=cluster{"Data":string[], "State":T1} {"Data"=["999"], "State"=enum."扫码回复"} ("元素"), timeout in ms (-1)=10 ("超时毫秒(-1)")) -> ()  [unwired: 1 in, 3 out]
              }
            }
            n355 = case shown="0, 默认" w4922 {
              tunnel: [cluster{"Data":string[], "State":T1} {"Data"=[], "State"=enum."读数据保存请求"} ("元素") w4949 w4951] -> w4921
              tunnel: w4913 -> [_ w4950 w4952]
              frame 0, Default {
              }
              frame 1 {
                w4949 = cluster{"Data":string[], "State":T1} {"Data"=[], "State"=enum."读二维码"} ("元素")
                n356 = Enqueue Element(queue=w4950, element=w4949, timeout in ms (-1)=10 ("超时毫秒(-1)")) -> ()  [unwired: 1 in, 3 out]
              }
              frame 2 {
                w4951 = cluster{"Data":string[], "State":T1} {"Data"=["999"], "State"=enum."扫码回复"} ("元素")
                n357 = Enqueue Element(queue=w4952, element=w4951, timeout in ms (-1)=10 ("超时毫秒(-1)")) -> ()  [unwired: 1 in, 3 out]
              }
            }
          }
          frame "读二维码" {
            w4969 = u16 0 items=["byte", "word", "Dword"] ("数据类型")
            w4965 = u8 132 items=["I/O (P)"=128, "Input (I)"=129, "Output (Q)"=130, "Bit Memory (M)"=131, "Data (DB)"=132, "Instance Data (DI)"=133, "Local Data (L)"=134, "Predecessor Local Data (VL)"=135] ("寄存器类型")
            n358 = call "S7_Read.vi"("TCP"=w4964, "DB #"=u16 20, "读取长度"=u16 17, "寄存器类型"=w4965, "起始地址"=u32 24, "数据类型"=w4969) -> ("TCP"=w4963:refnum<k5>, "数据"=w4970:u32[], "error out"=w4972:errorcluster)  [unwired: 6 in, 1 out]
            n359 = To Unsigned Word Integer(number=w4970) -> (unsigned 16bit integer=w4971:u16[])
            n360 = call "还原为字符串.vi"("error in (no error)"=w4972, "输入数组"=w4971) -> ("error out"=w4956:errorcluster, "字符串"=w4957:string)  [unwired: 8 in]
            n361 = Match Pattern(string=w4957, regular expression=" " ("正则表达式")) -> (before substring=w4954:string)  [unwired: 1 in, 3 out]
            n362 = flat-sequence {
              tunnel: w4956 -> [w4974]
              tunnel: [w4974] -> w4955
              tunnel: w4954 -> [w4973]
              tunnel: [w4977] -> w4960
              tunnel: w4955 -> [w4975]
              frame #0 {
                "502二维码" <- w4973
              }
              frame #1 {
                n363 = property on="ST502扫码请求(事件)" class="Bool (严格)"(error in=w4975, "Val(Sgnl)"=TRUE ("值(信号)")) -> (error out=w4977:errorcluster)  [unwired: 1 in, 1 out]
              }
            }
          }
          frame "扫码回复" {
            n364 = Array Size(array=w4982) -> (size(s)=w4981:i32)
            n365 = case shown="3, 默认" w4981 {
              tunnel: w4982 -> [w5012 w5021]
              tunnel: w4985 -> [w4999 w5022]
              tunnel: [w4990 w5024] -> w4984
              tunnel: [w4989 w5023] -> w4983
              tunnel: [w4988 w5020] -> w4980
              frame 3, Default {
                w5002 = u8 132 items=["I/O (P)"=128, "Input (I)"=129, "Output (Q)"=130, "Bit Memory (M)"=131, "Data (DB)"=132, "Instance Data (DI)"=133, "Local Data (L)"=134, "Predecessor Local Data (VL)"=135] ("寄存器类型")
                w5001 = u16 1 items=["byte", "word", "Dword"] ("数据类型")
                w5009 = u8 132 items=["I/O (P)"=128, "Input (I)"=129, "Output (Q)"=130, "Bit Memory (M)"=131, "Data (DB)"=132, "Instance Data (DI)"=133, "Local Data (L)"=134, "Predecessor Local Data (VL)"=135] ("寄存器类型")
                w5010 = u16 1 items=["byte", "word", "Dword"] ("数据类型")
                w5016 = u8 132 items=["I/O (P)"=128, "Input (I)"=129, "Output (Q)"=130, "Bit Memory (M)"=131, "Data (DB)"=132, "Instance Data (DI)"=133, "Local Data (L)"=134, "Predecessor Local Data (VL)"=135] ("寄存器类型")
                w5015 = u16 1 items=["byte", "word", "Dword"] ("数据类型")
                n366 = Index Array(array=w5012) -> (element #1=w4988:string, element #2=w4995:string, element #3=w4994:string)  [unwired: 3 in]
                n367 = Equal?(x=w4994, y="OK") -> (x = y?=w4992:bool)
                n368 = Decimal String To Number(string=w4995, default (0L)=u32 0 ("默认(0 I32)")) -> (number=w4996:u32)  [unwired: 1 in, 1 out]
                n369 = case shown="假" w4992 {
                  tunnel: [u32 2 ("写入数据") u32 1 ("写入数据")] -> w4991
                  frame False {
                  }
                  frame True {
                  }
                }
                n370 = call "S7_Write.vi"("TCP"=w4999, "寄存器类型"=w5016, "DB #"=u16 20, "写入地址"=u32 8, "数据类型"=w5015, "写入数据"=w4996) -> ("TCP"=w5006:refnum<k5>, "error out"=w5007:errorcluster)  [unwired: 7 in, 1 out]
                n371 = call "S7_Write.vi"("TCP"=w5006, "寄存器类型"=w5009, "DB #"=u16 20, "写入地址"=u32 10, "数据类型"=w5010, "写入数据"=w4991, "error in"=w5007) -> ("TCP"=w4998:refnum<k5>, "error out"=w4997:errorcluster)  [unwired: 6 in, 1 out]
                n372 = Decimal String To Number(string=w4988, default (0L)=u32 0 ("默认(0 I32)")) -> (number=w5005:u32)  [unwired: 1 in, 1 out]
                n373 = call "S7_Write.vi"("TCP"=w4998, "寄存器类型"=w5002, "DB #"=u16 20, "写入地址"=u32 2, "数据类型"=w5001, "写入数据"=w5005, "error in"=w4997) -> ("TCP"=w4990:refnum<k5>, "error out"=w4989:errorcluster)  [unwired: 6 in, 1 out]
              }
              frame 1 {
                w5027 = u8 132 items=["I/O (P)"=128, "Input (I)"=129, "Output (Q)"=130, "Bit Memory (M)"=131, "Data (DB)"=132, "Instance Data (DI)"=133, "Local Data (L)"=134, "Predecessor Local Data (VL)"=135] ("寄存器类型")
                w5026 = u16 1 items=["byte", "word", "Dword"] ("数据类型")
                n374 = Index Array(array=w5021) -> (element=w5020:string)  [unwired: 1 in]
                n375 = Decimal String To Number(string=w5020, default (0L)=u32 0 ("默认(0 I32)")) -> (number=w5030:u32)  [unwired: 1 in, 1 out]
                n376 = call "S7_Write.vi"("TCP"=w5022, "寄存器类型"=w5027, "DB #"=u16 20, "写入地址"=u32 2, "数据类型"=w5026, "写入数据"=w5030) -> ("TCP"=w5024:refnum<k5>, "error out"=w5023:errorcluster)  [unwired: 7 in, 1 out]
              }
            }
            "扫码请求回复501" <- w4980
            n377 = Bundle By Name(cluster=w4979, "扫码超时1"=w4980) -> (w4978:T7)
          }
          frame "-------------" {
          }
          frame "读数据保存请求" {
            w5064 = u16 0 items=["byte", "word", "Dword"] ("数据类型")
            w5066 = u8 132 items=["I/O (P)"=128, "Input (I)"=129, "Output (Q)"=130, "Bit Memory (M)"=131, "Data (DB)"=132, "Instance Data (DI)"=133, "Local Data (L)"=134, "Predecessor Local Data (VL)"=135] ("寄存器类型")
            n378 = call "S7_Read.vi"("TCP"=w5056, "DB #"=u16 20, "读取长度"=u16 1, "寄存器类型"=w5066, "起始地址"=u32 0, "数据类型"=w5064) -> ("TCP"=w5055:refnum<k5>, "数据"=w5061:u32[], "error out"=w5054:errorcluster)  [unwired: 6 in, 1 out]
            n379 = Index Array(array=w5061, index=0 ("索引")) -> (element=w5059:u32)
            n380 = Number To Boolean Array(number=w5059) -> (Boolean array=w5058:bool[])
            n381 = Unbundle By Name(w5037) -> ("数据保存超时1"=w5038:string)
            n382 = Index Array(array=w5058, index=1 ("索引")) -> (element=w5043:bool)
            "ST501数据读取" <- w5043
            n383 = Not Equal?(x=w5038, y="999") -> (x != y?=w5040:bool)
            n384 = Not(x=w5040) -> (.not. x?=w5041:bool)
            n385 = call <vilib>:"Boolean Crossing PtByPt.vi"("direction"=enum16{"either", "false-true", "true-false"}."false-true", "input"=w5043) -> ("crossing"=w5047:bool)  [unwired: 1 in]
            n386 = call <vilib>:"Boolean Crossing PtByPt.vi"("direction"=enum16{"either", "false-true", "true-false"}."true-false", "input"=w5043) -> ("crossing"=w5048:bool)  [unwired: 1 in]
            n387 = call "已用时间12"("Reset"=w5041) -> ("Time has Elapsed"=w5042:bool)  [unwired: 11 in, 7 out]
            n388 = Insert Into Array(array=bool[] [] ("数组"), index=0 ("索引"), new element #1=w5047, new element #2=w5048) -> (w5051:bool[])
            n389 = Boolean Array To Number(Boolean array=w5051) -> (number=w5052:u32)
            n390 = case shown="2" w5052 {
              tunnel: [cluster{"Data":string[], "State":T1} {"Data"=[], "State"=enum."读扫码请求2"} ("元素") w5071 w5075] -> w5044
              tunnel: w5036 -> [_ w5072 w5076]
              frame 0, Default {
              }
              frame 1 {
                w5071 = cluster{"Data":string[], "State":T1} {"Data"=[], "State"=enum."读数据"} ("元素")
                n391 = Enqueue Element(queue=w5072, element=w5071, timeout in ms (-1)=10 ("超时毫秒(-1)")) -> ()  [unwired: 1 in, 3 out]
              }
              frame 2 {
                w5075 = cluster{"Data":string[], "State":T1} {"Data"=["999"], "State"=enum."数据保存回复"} ("元素")
                n392 = Enqueue Element(queue=w5076, element=w5075, timeout in ms (-1)=10 ("超时毫秒(-1)")) -> ()  [unwired: 1 in, 3 out]
              }
            }
            n393 = case shown="真" w5042 {
              tunnel: w5036 -> [_ w5068]
              frame False {
              }
              frame True {
                n394 = Enqueue Element(queue=w5068, element=cluster{"Data":string[], "State":T1} {"Data"=["999"], "State"=enum."数据保存回复"} ("元素"), timeout in ms (-1)=10 ("超时毫秒(-1)")) -> ()  [unwired: 1 in, 3 out]
              }
            }
          }
          frame "读数据" {
            w5090 = u16 2 items=["byte", "word", "Dword"] ("数据类型")
            w5088 = u8 132 items=["I/O (P)"=128, "Input (I)"=129, "Output (Q)"=130, "Bit Memory (M)"=131, "Data (DB)"=132, "Instance Data (DI)"=133, "Local Data (L)"=134, "Predecessor Local Data (VL)"=135] ("寄存器类型")
            w5098 = u16 0 items=["byte", "word", "Dword"] ("数据类型")
            w5100 = u8 132 items=["I/O (P)"=128, "Input (I)"=129, "Output (Q)"=130, "Bit Memory (M)"=131, "Data (DB)"=132, "Instance Data (DI)"=133, "Local Data (L)"=134, "Predecessor Local Data (VL)"=135] ("寄存器类型")
            w5136 = u16 1 items=["byte", "word", "Dword"] ("数据类型")
            w5132 = u8 132 items=["I/O (P)"=128, "Input (I)"=129, "Output (Q)"=130, "Bit Memory (M)"=131, "Data (DB)"=132, "Instance Data (DI)"=133, "Local Data (L)"=134, "Predecessor Local Data (VL)"=135] ("寄存器类型")
            n395 = call "S7_Read.vi"("TCP"=w5097, "DB #"=u16 20, "读取长度"=u16 1, "寄存器类型"=w5100, "起始地址"=u32 0, "数据类型"=w5098) -> ("TCP"=w5086:refnum<k5>, "数据"=w5106:u32[], "error out"=w5085:errorcluster)  [unwired: 6 in, 1 out]
            n396 = Index Array(array=w5106, index=0 ("索引")) -> (element=w5104:u32)
            n397 = Number To Boolean Array(number=w5104) -> (Boolean array=w5103:bool[])
            n398 = Index Array(array=w5103, index=4 ("索引")) -> (element=w5093:bool)
            n399 = call "S7_Read.vi"("TCP"=w5086, "DB #"=u16 20, "读取长度"=u16 2, "寄存器类型"=w5088, "起始地址"=u32 180, "数据类型"=w5090, "error in"=w5085) -> ("TCP"=w5084:refnum<k5>, "数据"=w5081:u32[], "error out"=w5083:errorcluster)  [unwired: 5 in, 1 out]
            n400 = Equal?(x=w5093, y=TRUE) -> (x = y?=w5095:bool)
            n401 = Index Array(array=w5081, index #1=0 ("索引")) -> (element #1=w5080:u32, element #2=w5079:u32)  [unwired: 1 in]
            n402 = case shown="假" w5095 {
              tunnel: [" " "Y"] -> w5092
              frame False {
              }
              frame True {
              }
            }
            n403 = Number To Decimal String(number=w5080) -> (decimal integer string=w5078:string)  [unwired: 1 in]
            n404 = Number To Decimal String(number=w5079) -> (decimal integer string=w5077:string)  [unwired: 1 in]
            n405 = local read "ST502 Pressure Plate M0105053"() -> (w5107:string)
            n406 = local read "ST502 Support Ring 5027083"() -> (w5109:string)
            n407 = call "S7_Read.vi"("TCP"=w5084, "DB #"=u16 20, "读取长度"=u16 1, "寄存器类型"=w5132, "起始地址"=u32 6, "数据类型"=w5136, "error in"=w5083) -> ("TCP"=w5118:refnum<k5>, "数据"=w5131:u32[], "error out"=w5121:errorcluster)  [unwired: 5 in, 1 out]
            n408 = local read "ST502 Form Seal 5026860"() -> (w5110:string)
            n409 = local read "ST502 O-Ring M0104976"() -> (w5108:string)
            n410 = Index Array(array=w5131) -> (element=w5120:u32)  [unwired: 1 in]
            n411 = Equal?(x=w5120, y=u32 1) -> (x = y?=w5129:bool)
            n412 = case shown="假" w5129 {
              tunnel: ["NG" "OK"] -> w5119
              frame False {
              }
              frame True {
              }
            }
            n413 = Format Date/Time String(time format string (%c)="%Y-%m-%d" ("时间格式字符串(%c)")) -> (date/time string=w5123:string)  [unwired: 2 in]
            n414 = Get Date/Time String() -> (time string=w5122:string)  [unwired: 3 in, 1 out]
            n415 = Insert Into Array(array=string[] [] ("数组"), index=0 ("索引"), new element #1="502" ("新元素/子数组"), new element #2=w5119, new element #3=w5123, new element #4=w5122, new element #5=w5119, new element #6=w5110, new element #7=w5109, new element #8=w5108, new element #9=w5107, new element #10=w5092, new element #11=w5078, new element #12=w5077) -> (w5128:string[])
            n416 = Enqueue Element(queue=w5117, element=w5128, error in (no error)=w5121) -> (error out=w5111:errorcluster)  [unwired: 1 in, 2 out]
            n417 = property on="ST502数据读取（事件）" class="Bool (严格)"(error in=w5111, "Val(Sgnl)"=TRUE ("值(信号)")) -> (error out=w5112:errorcluster)  [unwired: 1 in, 1 out]
          }
          frame "数据保存回复" {
            w5154 = u8 132 items=["I/O (P)"=128, "Input (I)"=129, "Output (Q)"=130, "Bit Memory (M)"=131, "Data (DB)"=132, "Instance Data (DI)"=133, "Local Data (L)"=134, "Predecessor Local Data (VL)"=135] ("寄存器类型")
            w5155 = u16 1 items=["byte", "word", "Dword"] ("数据类型")
            n418 = Index Array(array=w5148, index=0 ("索引")) -> (element=w5141:string)
            "数据保存请求回复501" <- w5141
            n419 = Decimal String To Number(string=w5141, default (0L)=u32 0 ("默认(0 I32)")) -> (number=w5150:u32)  [unwired: 1 in, 1 out]
            n420 = call "S7_Write.vi"("TCP"=w5149, "寄存器类型"=w5154, "DB #"=u16 20, "写入地址"=u32 4, "数据类型"=w5155, "写入数据"=w5150) -> ("TCP"=w5146:refnum<k5>, "error out"=w5147:errorcluster)  [unwired: 7 in, 1 out]
            n421 = Bundle By Name(cluster=w5143, "数据保存超时1"=w5141) -> (w5142:T7)
          }
          frame "-----------------" {
          }
          frame "错误" {
            n422 = Flush Queue(queue=w5164) -> ()  [unwired: 1 in, 3 out]
            n423 = Flush Queue(queue=w5163) -> ()  [unwired: 1 in, 3 out]
            n424 = call "S7_Close.vi"("TCP Connection Ref"=w5167) -> ("error out"=w5165:errorcluster)  [unwired: 10 in]
            n425 = call <vilib>:"Clear Errors.vi"("error in (no error)"=w5165) -> ()  [unwired: 5 in, 2 out]
          }
          frame "退出" {
            n426 = Release Queue(queue=w5176) -> ()  [unwired: 2 in, 3 out]
            n427 = Release Queue(queue=w5175) -> ()  [unwired: 2 in, 3 out]
            n428 = call "S7_Close.vi"("TCP Connection Ref"=w5174) -> ("error out"=w5173:errorcluster)  [unwired: 10 in]
          }
          frame "-------------------" {
          }
          frame "读扫码请求2" {
            w5197 = u8 132 items=["I/O (P)"=128, "Input (I)"=129, "Output (Q)"=130, "Bit Memory (M)"=131, "Data (DB)"=132, "Instance Data (DI)"=133, "Local Data (L)"=134, "Predecessor Local Data (VL)"=135] ("寄存器类型")
            w5196 = u16 1 items=["byte", "word", "Dword"] ("数据类型")
            w5225 = u16 0 items=["byte", "word", "Dword"] ("数据类型")
            w5227 = u8 132 items=["I/O (P)"=128, "Input (I)"=129, "Output (Q)"=130, "Bit Memory (M)"=131, "Data (DB)"=132, "Instance Data (DI)"=133, "Local Data (L)"=134, "Predecessor Local Data (VL)"=135] ("寄存器类型")
            n429 = Unbundle By Name(w5188) -> ("看门狗"=w5194:string)
            n430 = Decimal String To Number(string=w5194) -> (number=w5193:i32)  [unwired: 2 in, 1 out]
            n431 = Equal?(x=w5193, y=0) -> (x = y?=w5191:bool)
            n432 = case shown="假" w5191 {
              tunnel: [0 ("y") 1 ("y")] -> w5189
              frame False {
              }
              frame True {
              }
            }
            n433 = call "S7_Write.vi"("TCP"=w5186, "寄存器类型"=w5197, "DB #"=u16 20, "写入地址"=u32 22, "数据类型"=w5196, "写入数据"=w5189) -> ("TCP"=w5185:refnum<k5>, "error out"=w5184:errorcluster)  [unwired: 7 in, 1 out]
            n434 = Number To Decimal String(number=w5189) -> (decimal integer string=w5190:string)  [unwired: 1 in]
            n435 = local write "50"(w5189) -> ()
            n436 = Bundle By Name(cluster=w5188, "看门狗"=w5190) -> (w5187:T7)
